vi "Omniax_mDrive_COM8_COM9.vi"() -> ()   [LabVIEW 2009]
uses:
  <vilib>/Instr/_visa.llb/VISA Configure Serial Port (Instr).vi
panel:
  in  "GPIT Backlash":i32
  in  "DETT Backlash":i32
  in  "SY/SZ":dbl max=1.0 step=1.0
  out "GPIT Status":string
  out "read buffer 3":string
  out "SZ":i32
  out "SZ Range?":bool
  out "GPIT rev/sec":dbl caption="Velocity"
  out "GPIT MINPOS":i32=-94296
  out "GPIT MAXPOS":i32=-34296
  out "GPIT COM PORT":refnum<visa-resource-name>="COM5"
  out "SZ Step":i32
  in  "Stop":bool
  out "SY Range?":bool
  out "SY":i32
  out "read buffer 2":string
  out "DETH Status":string
  out "DETH rev//sec":dbl caption="Velocity"
  in  "Go":bool
  in  "SY Step":i32=-1000 min=-1000 max=1000 step=100
  out "DETH MINPOS":i32=-94296
  out "DETH MAXPOS":i32=-34296
  out "DETT COM PORT":refnum<visa-resource-name>="COM5"
  # "SY COM8 & SZ COM9"
  # "20000 steps/rev\n2.5mm/rev\n0.05rev/sec"
  # "20000 steps/rev\n1 mm/rev\n0.01rev/sec"
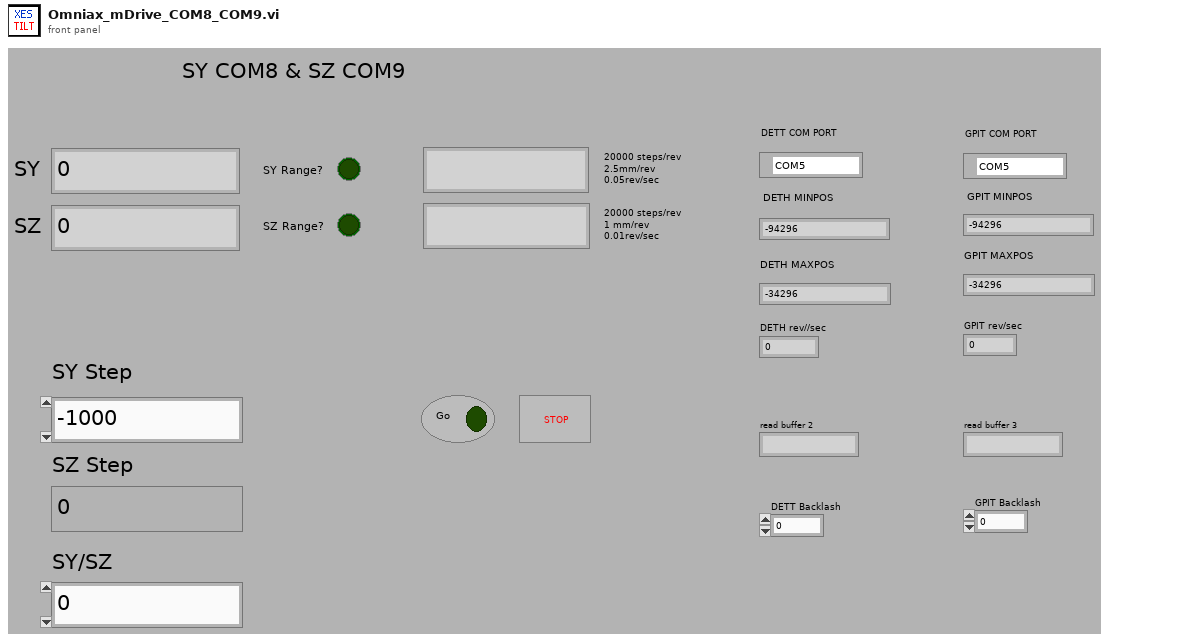
[diagram p1: front panel]
types:
  T1 = enum16{"Stop", "Reset", "Run Current", "Holding Current", "Accel Rate", "Decel Rate", "Move to Relative Position", "Move to Absolute Position", "Prtint Position", "Print Encorder", "Print Velocity", "Microstep Resolution", "Max Velocity"}
  T2 = enum16{"Power-up Signature", "Accel Rate", "Accel Max", "Bit Rate", "Buffer Status", "Change Current", "Commence Jogging", "Change Jog Speed", "Continue", "Define Address", "Distance for FC,FM,FO,FY", "Decel Rate", "Distance or Position", "Define Limits", "Encoder Deadband", "Encoder Function", "Encoder Position", "Encoder Ratio", "Feed to Length with Speed Change", "Feed to Length", "Feed to Sensor with Mask Dist", "Feed to Length & Set Output", "Feed to Position", "Feed to Sensor", "Feed to Sensor w/safety", "Follow Handwheel", "Immediate Distance?", "Immediate Encoder?", "Immediate Low Output", "Immediate High Output", "Immediate Position?", "Input Status?", "Jog Accel/Decel", "Jog Disable", "Jog Enable", "Jog Speed", "Motor Disable", "Motor Enable", "Microstep Resolution", "Power up Current", "Power up Mode", "Pause", "Request Status", "Revision Level?", "Seek Home", "Stop Jogging", "Stop & Kill Buffer", "Set Output", "Set ABS Position", "Send String", "Stop", "Velocity for Speed Change", "Velocity Setting", "Wait for Input", "Wait Time"}
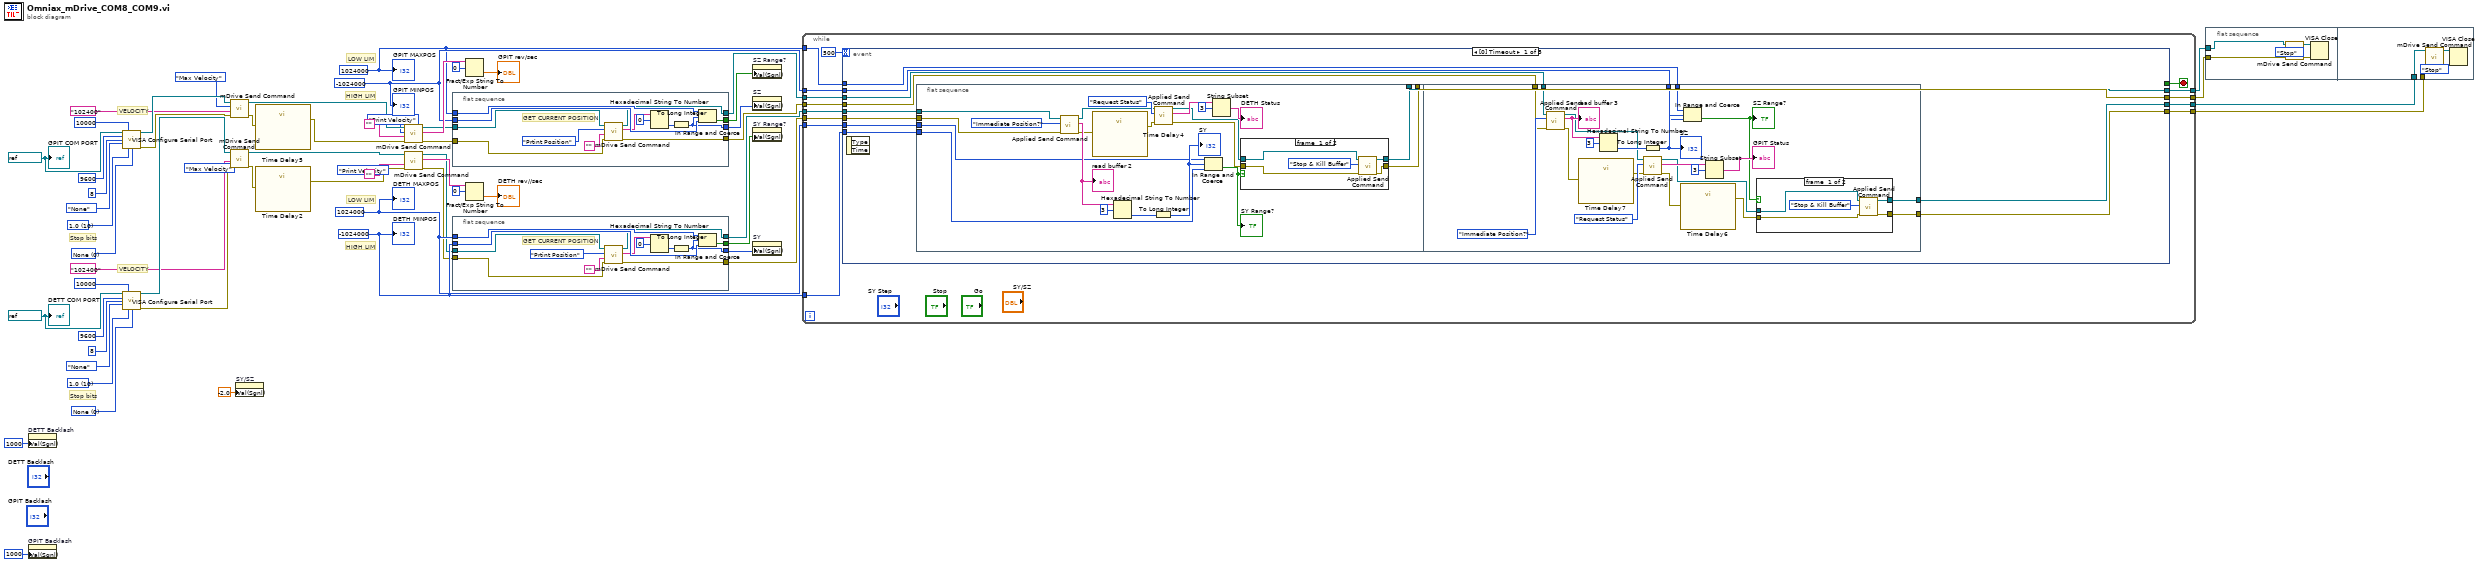
[diagram p0: block diagram]
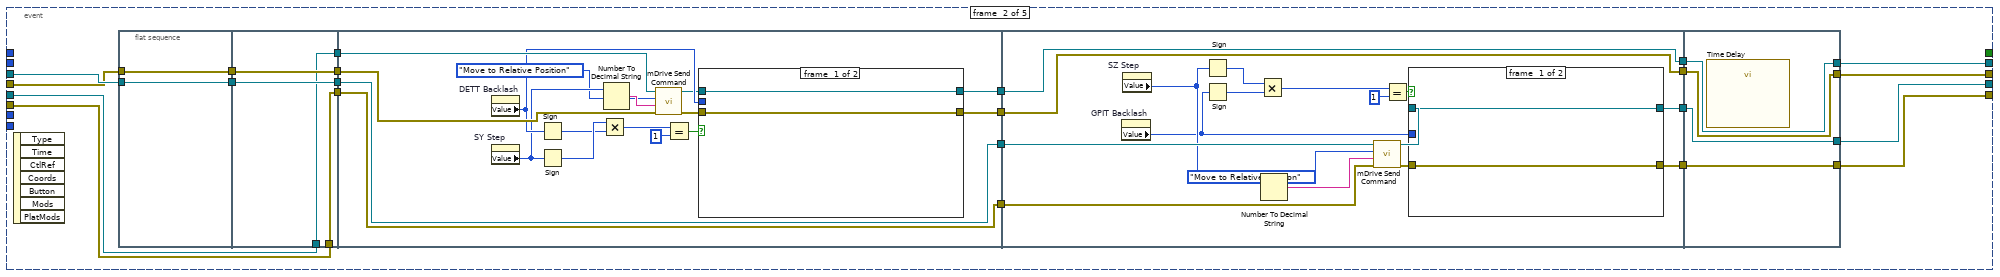
[diagram p4: hidden frame]
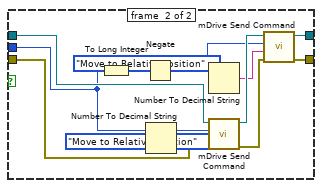
[diagram p5: hidden frame]
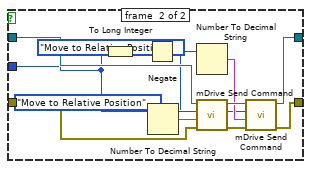
[diagram p6: hidden frame]
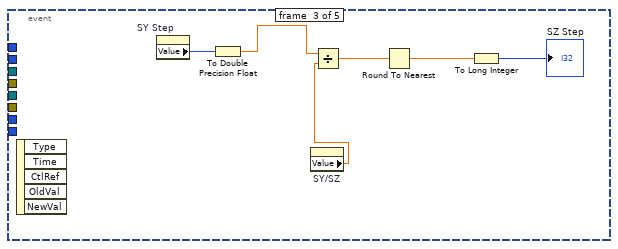
[diagram p7: hidden frame]
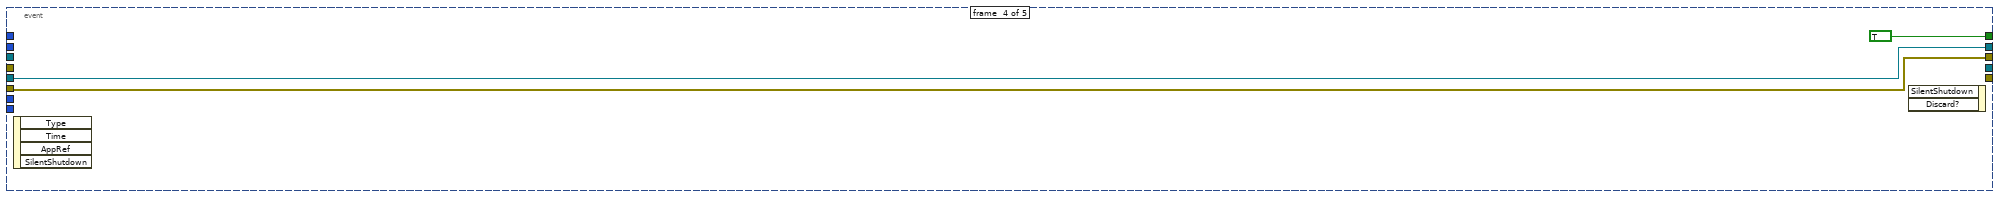
[diagram p8: hidden frame]
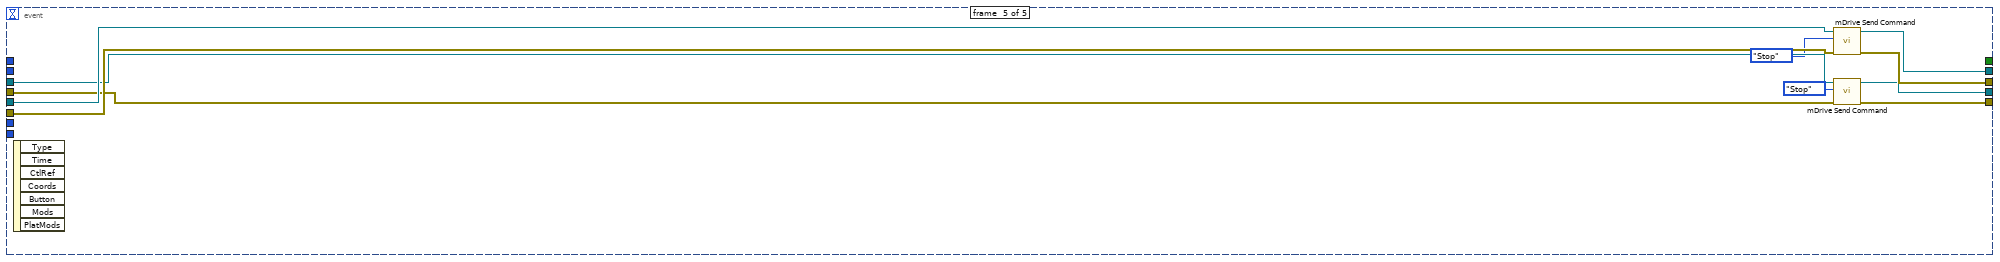
[diagram p9: hidden frame]
diagram:
  w16 = -1024000 ("lower limit")
  w15 = 1024000 ("upper limit")
  w29 = refnum<visa-resource-name> "COM8" ("COM PORT")
  w31 = u16 0 items=["None", "XON/XOFF", "RTS/CTS", "XON/XOFF & RTS/CTS", "DTR/DSR", "XON/XOFF & DTR/DSR"] ("flow control (0:none)")
  w32 = u16 10 items=["1.0"=10, "1.5"=15, "2.0"=20] ("stop bits (10: 1 bit)")
  w51 = -1024000 ("lower limit")
  w52 = 1024000 ("upper limit")
  w55 = refnum<visa-resource-name> "COM9" ("COM PORT")
  w57 = u16 0 items=["None", "XON/XOFF", "RTS/CTS", "XON/XOFF & RTS/CTS", "DTR/DSR", "XON/XOFF & DTR/DSR"] ("flow control (0:none)")
  w58 = u16 10 items=["1.0"=10, "1.5"=15, "2.0"=20] ("stop bits (10: 1 bit)")
  # "VELOCITY"
  # "HIGH LIM"
  # "LOW LIM"
  # "Stop bits"
  # "VELOCITY"
  # "HIGH LIM"
  # "LOW LIM"
  # "Stop bits"
  n1 = property on="DETT Backlash" class="DigNum (strict)"("Val(Sgnl)"=1000 ("Value (Signaling)")) -> ()  [unwired: 2 in, 2 out]
  n2 = property on="GPIT Backlash" class="DigNum (strict)"("Val(Sgnl)"=1000 ("Value (Signaling)")) -> ()  [unwired: 2 in, 2 out]
  n3 = call-poly "VISA Configure Serial Port"("VISA resource name"=w29, "timeout (10sec)"=u32 10000, "baud rate (9600)"=u32 9600, "data bits (8)"=u16 8, "parity (0:none)"=enum16{"None", "Odd", "Even", "Mark", "Space"}."None", "stop bits (10: 1 bit)"=w32, "flow control (0:none)"=w31) -> ("VISA resource name out"=w19:refnum<visa-resource-name>, "error out"=w18:errorcluster)  [unwired: 7 in]
  n4 = call-poly "VISA Configure Serial Port"("VISA resource name"=w55, "timeout (10sec)"=u32 10000, "baud rate (9600)"=u32 9600, "data bits (8)"=u16 8, "parity (0:none)"=enum16{"None", "Odd", "Even", "Mark", "Space"}."None", "stop bits (10: 1 bit)"=w58, "flow control (0:none)"=w57) -> ("VISA resource name out"=w39:refnum<visa-resource-name>, "error out"=w38:errorcluster)  [unwired: 7 in]
  n5 = call "mDrive Send Command.vi"("error in (no error)"=w18, "Extra"="102400", "Command"=T1."Max Velocity", "VISA resource name"=w19) -> ("error out"=w28:errorcluster, "VISA resource name out"=w24:refnum<visa-resource-name>)  [unwired: 3 in, 1 out]
  n6 = call "mDrive Send Command.vi"("error in (no error)"=w38, "Extra"="102400", "Command"=T1."Max Velocity", "VISA resource name"=w39) -> ("error out"=w50:errorcluster, "VISA resource name out"=w46:refnum<visa-resource-name>)  [unwired: 3 in, 1 out]
  n7 = property on="SY/SZ" class="DigNum (strict)"("Val(Sgnl)"=-2.0 ("Value (Signaling)")) -> ()  [unwired: 2 in, 2 out]
  n8 = call "Time Delay5"("error in (no error)"=w28) -> ("error out"=w25:errorcluster)  [unwired: 10 in]
  n9 = call "Time Delay2"("error in (no error)"=w50) -> ("error out"=w47:errorcluster)  [unwired: 10 in]
  n10 = call "mDrive Send Command.vi"("error in (no error)"=w25, "Extra"="", "Command"=T1."Print Velocity", "VISA resource name"=w24) -> ("error out"=w22:errorcluster, "read buffer"=w27:string, "VISA resource name out"=w23:refnum<visa-resource-name>)  [unwired: 3 in]
  n11 = call "mDrive Send Command.vi"("error in (no error)"=w47, "Extra"="", "Command"=T1."Print Velocity", "VISA resource name"=w46) -> ("error out"=w44:errorcluster, "read buffer"=w49:string, "VISA resource name out"=w45:refnum<visa-resource-name>)  [unwired: 3 in]
  n12 = flat-sequence {
    tunnel: w22 -> [w74]
    tunnel: w23 -> [w73]
    tunnel: w15 -> [w71]
    tunnel: w16 -> [w70]
    tunnel: [w72] -> w13
    tunnel: [w63] -> w8
    tunnel: [w69] -> w10
    tunnel: [w68] -> w14
    frame #0 {
      # "GET CURRENT POSITION"
      n13 = call "mDrive Send Command.vi"("error in (no error)"=w74, "Extra"="", "Command"=T1."Prtint Position", "VISA resource name"=w73) -> ("error out"=w72:errorcluster, "read buffer"=w66:string, "VISA resource name out"=w68:refnum<visa-resource-name>)  [unwired: 3 in]
      n14 = Hexadecimal String To Number(string=w66, offset=0) -> (number=w64:u32)  [unwired: 1 in, 1 out]
      n15 = To Long Integer(number=w64) -> (32bit integer=w63:i32)
      n16 = In Range and Coerce(upper limit=w71, x=w63, lower limit=w70) -> (In Range?=w69:bool)  [unwired: 1 out]
    }
  }
  n17 = flat-sequence {
    tunnel: w44 -> [w87]
    tunnel: w45 -> [w86]
    tunnel: w52 -> [w85]
    tunnel: w51 -> [w84]
    tunnel: [w76] -> w53
    tunnel: [w77] -> w9
    tunnel: [w83] -> w36
    tunnel: [w82] -> w54
    frame #0 {
      # "GET CURRENT POSITION"
      n18 = call "mDrive Send Command.vi"("error in (no error)"=w87, "Extra"="", "Command"=T1."Prtint Position", "VISA resource name"=w86) -> ("error out"=w76:errorcluster, "read buffer"=w80:string, "VISA resource name out"=w82:refnum<visa-resource-name>)  [unwired: 3 in]
      n19 = Hexadecimal String To Number(string=w80, offset=0) -> (number=w78:u32)  [unwired: 1 in, 1 out]
      n20 = To Long Integer(number=w78) -> (32bit integer=w77:i32)
      n21 = In Range and Coerce(upper limit=w85, x=w77, lower limit=w84) -> (In Range?=w83:bool)  [unwired: 1 out]
    }
  }
  n22 = Fract/Exp String To Number(string=w27, offset=0) -> (number=→"GPIT rev/sec":dbl)  [unwired: 2 in, 1 out]
  n23 = Fract/Exp String To Number(string=w49, offset=0) -> (number=→"DETH rev//sec":dbl)  [unwired: 2 in, 1 out]
  n24 = property on="SZ Range?" class="Bool (strict)"("Val(Sgnl)"=w10) -> ()  [unwired: 2 in, 2 out]
  n25 = property on="SZ" class="DigNum (strict)"("Val(Sgnl)"=w8) -> ()  [unwired: 2 in, 2 out]
  n26 = property on="SY Range?" class="Bool (strict)"("Val(Sgnl)"=w36) -> ()  [unwired: 2 in, 2 out]
  n27 = property on="SY" class="DigNum (strict)"("Val(Sgnl)"=w9) -> ()  [unwired: 2 in, 2 out]
  n28 = while {
    tunnel: w54 -> [w95]
    tunnel: w53 -> [w100]
    tunnel: [w101] -> w40
    tunnel: [w99] -> w41
    tunnel: w52 -> [w98]
    tunnel: w51 -> [w97]
    tunnel: w16 -> [w93]
    tunnel: w15 -> [w88]
    tunnel: w14 -> [w92]
    tunnel: w13 -> [w91]
    tunnel: [w90] -> w12
    tunnel: [w89] -> w11
    stop <- w94 stop-if-true
    n29 = event shown="[0] Timeout" {
      selector: _ -> [_ _ _ _ _]
      dyn-events: _ -> [_ _ _ _ _]
      timeout: 500 -> [_ _ _ _ _]
      tunnel: w100 -> [w111 w172 _ w274 w284]
      tunnel: [w105 w179 _ w274 w282] -> w101
      tunnel: w95 -> [w110 w171 _ w275 w285]
      tunnel: [w104 w192 _ w275 w283] -> w99
      tunnel: w98 -> [w113 _ _ _ _]
      tunnel: w97 -> [w112 _ _ _ _]
      tunnel: [_ _ _ TRUE _] -> w94
      tunnel: w93 -> [w102 _ _ _ _]
      tunnel: w88 -> [w103 _ _ _ _]
      tunnel: w92 -> [w109 w187 _ _ w279]
      tunnel: w91 -> [w108 w183 _ _ w278]
      tunnel: [w107 w177 _ _ w281] -> w90
      tunnel: [w106 w175 _ _ w280] -> w89
      event #0 {
        n30 = event-data() -> ()  [unwired: 1 in, 2 out]
        n31 = flat-sequence {
          tunnel: w112 -> [w134]
          tunnel: w113 -> [w126]
          tunnel: w111 -> [w125]
          tunnel: w110 -> [w124]
          tunnel: [w116] -> w104
          tunnel: [w114] -> w105
          tunnel: w109 -> [w150]
          tunnel: w108 -> [w149]
          tunnel: w103 -> [w148]
          tunnel: w102 -> [w147]
          tunnel: [w144] -> w107
          tunnel: [w145] -> w106
          frame #0 {
            n32 = call "Applied Send Command.vi"("error in (no error)"=w125, "Command"=T2."Immediate Position?", "VISA resource name"=w124) -> ("error out"=w120:errorcluster, "read buffer"=w132:string, "VISA resource name out"=w127:refnum<visa-resource-name>)  [unwired: 4 in]
            "read buffer 2" <- w132
            n33 = call "Time Delay4"("error in (no error)"=w120) -> ("error out"=w119:errorcluster)  [unwired: 10 in]
            n34 = Hexadecimal String To Number(string=w132, offset=3) -> (number=w131:u32)  [unwired: 1 in, 1 out]
            n35 = call "Applied Send Command.vi"("error in (no error)"=w119, "Command"=T2."Request Status", "VISA resource name"=w127) -> ("error out"=w115:errorcluster, "read buffer"=w123:string, "VISA resource name out"=w117:refnum<visa-resource-name>)  [unwired: 4 in]
            n36 = To Long Integer(number=w131) -> (32bit integer=w129:i32)
            "SY" <- w129
            n37 = In Range and Coerce(upper limit=w126, x=w129, lower limit=w134) -> (In Range?=w118:bool)  [unwired: 1 out]
            "SY Range?" <- w118
            n38 = String Subset(string=w123, offset (0)=3) -> (substring=→"DETH Status":string)  [unwired: 1 in]
            n39 = case shown="False" w118 {
              tunnel: w117 -> [w136 w141]
              tunnel: [w138 w141] -> w116
              tunnel: [w139 w140] -> w114
              tunnel: w115 -> [w135 w140]
              frame #0 {
                n40 = call "Applied Send Command.vi"("error in (no error)"=w135, "Command"=T2."Stop & Kill Buffer", "VISA resource name"=w136) -> ("error out"=w139:errorcluster, "VISA resource name out"=w138:refnum<visa-resource-name>)  [unwired: 4 in, 1 out]
              }
              frame #1 {
              }
            }
          }
          frame #1 {
            n41 = call "Applied Send Command.vi"("error in (no error)"=w149, "Command"=T2."Immediate Position?", "VISA resource name"=w150) -> ("error out"=w152:errorcluster, "read buffer"=w162:string, "VISA resource name out"=w157:refnum<visa-resource-name>)  [unwired: 4 in]
            "read buffer 3" <- w162
            n42 = call "Time Delay7"("error in (no error)"=w152) -> ("error out"=w151:errorcluster)  [unwired: 10 in]
            n43 = Hexadecimal String To Number(string=w162, offset=3) -> (number=w161:u32)  [unwired: 1 in, 1 out]
            n44 = To Long Integer(number=w161) -> (32bit integer=w159:i32)
            "SZ" <- w159
            n45 = call "Applied Send Command.vi"("error in (no error)"=w151, "Command"=T2."Request Status", "VISA resource name"=w157) -> ("error out"=w156:errorcluster, "read buffer"=w155:string, "VISA resource name out"=w143:refnum<visa-resource-name>)  [unwired: 4 in]
            n46 = call "Time Delay6"("error in (no error)"=w156) -> ("error out"=w146:errorcluster)  [unwired: 10 in]
            n47 = In Range and Coerce(upper limit=w148, x=w159, lower limit=w147) -> (In Range?=w142:bool)  [unwired: 1 out]
            "SZ Range?" <- w142
            n48 = String Subset(string=w155, offset (0)=3) -> (substring=→"GPIT Status":string)  [unwired: 1 in]
            n49 = case shown="False" w142 {
              tunnel: w143 -> [w165 w170]
              tunnel: [w167 w170] -> w144
              tunnel: [w168 w169] -> w145
              tunnel: w146 -> [w164 w169]
              frame #0 {
                n50 = call "Applied Send Command.vi"("error in (no error)"=w164, "Command"=T2."Stop & Kill Buffer", "VISA resource name"=w165) -> ("error out"=w168:errorcluster, "VISA resource name out"=w167:refnum<visa-resource-name>)  [unwired: 4 in, 1 out]
              }
              frame #1 {
              }
            }
          }
        }
      }
      event #1 {
        n51 = event-data() -> ()  [unwired: 1 in, 7 out]
        n52 = flat-sequence {
          tunnel: w187 -> [w194]
          tunnel: [w194] -> w186
          tunnel: [w193] -> w184
          tunnel: w183 -> [w193]
          tunnel: [w198] -> w189
          tunnel: w186 -> [w198]
          tunnel: [w197] -> w185
          tunnel: w184 -> [w197]
          tunnel: [w196] -> w174
          tunnel: [w195] -> w173
          tunnel: w172 -> [w195]
          tunnel: w171 -> [w196]
          tunnel: [w201] -> w191
          tunnel: w189 -> [w215]
          tunnel: [w215] -> w188
          tunnel: w185 -> [w213]
          tunnel: [w212] -> w182
          tunnel: [w200] -> w181
          tunnel: w174 -> [w214]
          tunnel: w173 -> [w212]
          tunnel: w191 -> [w247]
          tunnel: [w247] -> w190
          tunnel: w188 -> [w246]
          tunnel: w182 -> [w245]
          tunnel: w181 -> [w244]
          tunnel: [w244] -> w180
          tunnel: [w232] -> w178
          tunnel: [w234] -> w176
          tunnel: [w266] -> w192
          tunnel: w190 -> [w266]
          tunnel: w180 -> [w265]
          tunnel: [w265] -> w179
          tunnel: w178 -> [w264]
          tunnel: [w264] -> w177
          tunnel: [w263] -> w175
          tunnel: w176 -> [w263]
          frame #0 {
          }
          frame #1 {
          }
          frame #2 {
            n53 = property on="DETT Backlash" class="DigNum (strict)"() -> ("Value"=w205:i32)  [unwired: 2 in, 2 out]
            n54 = property on="SY Step" class="DigNum (strict)"() -> ("Value"=w204:i32)  [unwired: 2 in, 2 out]
            n55 = Sign(1:w205) -> (0:w209:i32)
            n56 = Sign(1:w204) -> (0:w210:i32)
            n57 = Multiply(x=w210, y=w209) -> (x*y=w208:i32)
            n58 = Number To Decimal String(number=w204) -> (decimal integer string=w211:string)  [unwired: 1 in]
            n59 = call "mDrive Send Command.vi"("error in (no error)"=w213, "Extra"=w211, "Command"=T1."Move to Relative Position", "VISA resource name"=w214) -> ("error out"=w202:errorcluster, "VISA resource name out"=w203:refnum<visa-resource-name>)  [unwired: 3 in, 1 out]
            n60 = Equal?(x=w208, y=1) -> (x = y?=w206:bool)
            n61 = case shown="True" w206 {
              tunnel: w203 -> [w217 w230]
              tunnel: [w217 w224] -> w201
              tunnel: [w216 w225] -> w200
              tunnel: w202 -> [w216 w229]
              tunnel: w205 -> [_ w220]
              frame #0 {
              }
              frame #1 {
                n62 = To Long Integer(number=w220) -> (32bit integer=w222:i32)
                n63 = Negate(x=w222) -> (-x=w223:i32)
                n64 = Number To Decimal String(number=w220) -> (decimal integer string=w228:string)  [unwired: 1 in]
                n65 = Number To Decimal String(number=w223) -> (decimal integer string=w221:string)  [unwired: 1 in]
                n66 = call "mDrive Send Command.vi"("error in (no error)"=w229, "Extra"=w228, "Command"=T1."Move to Relative Position", "VISA resource name"=w230) -> ("error out"=w226:errorcluster, "VISA resource name out"=w227:refnum<visa-resource-name>)  [unwired: 3 in, 1 out]
                n67 = call "mDrive Send Command.vi"("error in (no error)"=w226, "Extra"=w221, "Command"=T1."Move to Relative Position", "VISA resource name"=w227) -> ("error out"=w225:errorcluster, "VISA resource name out"=w224:refnum<visa-resource-name>)  [unwired: 3 in, 1 out]
              }
            }
          }
          frame #3 {
            n68 = property on="GPIT Backlash" class="DigNum (strict)"() -> ("Value"=w236:i32)  [unwired: 2 in, 2 out]
            n69 = property on="SZ Step" class="DigNum (strict)"() -> ("Value"=w238:i32)  [unwired: 2 in, 2 out]
            n70 = Sign(1:w238) -> (0:w242:i32)
            n71 = Sign(1:w236) -> (0:w241:i32)
            n72 = Multiply(x=w242, y=w241) -> (x*y=w240:i32)
            n73 = Number To Decimal String(number=w238) -> (decimal integer string=w243:string)  [unwired: 1 in]
            n74 = call "mDrive Send Command.vi"("error in (no error)"=w245, "Extra"=w243, "Command"=T1."Move to Relative Position", "VISA resource name"=w246) -> ("error out"=w235:errorcluster, "VISA resource name out"=w233:refnum<visa-resource-name>)  [unwired: 3 in, 1 out]
            n75 = Equal?(x=w240, y=1) -> (x = y?=w237:bool)
            n76 = case shown="True" w237 {
              tunnel: w233 -> [w249 w262]
              tunnel: [w249 w256] -> w232
              tunnel: [w248 w257] -> w234
              tunnel: w235 -> [w248 w261]
              tunnel: w236 -> [_ w252]
              frame #0 {
              }
              frame #1 {
                n77 = To Long Integer(number=w252) -> (32bit integer=w254:i32)
                n78 = Negate(x=w254) -> (-x=w255:i32)
                n79 = Number To Decimal String(number=w252) -> (decimal integer string=w260:string)  [unwired: 1 in]
                n80 = Number To Decimal String(number=w255) -> (decimal integer string=w253:string)  [unwired: 1 in]
                n81 = call "mDrive Send Command.vi"("error in (no error)"=w261, "Extra"=w260, "Command"=T1."Move to Relative Position", "VISA resource name"=w262) -> ("error out"=w258:errorcluster, "VISA resource name out"=w259:refnum<visa-resource-name>)  [unwired: 3 in, 1 out]
                n82 = call "mDrive Send Command.vi"("error in (no error)"=w258, "Extra"=w253, "Command"=T1."Move to Relative Position", "VISA resource name"=w259) -> ("error out"=w257:errorcluster, "VISA resource name out"=w256:refnum<visa-resource-name>)  [unwired: 3 in, 1 out]
              }
            }
          }
          frame #4 {
            n83 = call "Time Delay"() -> ()  [unwired: 11 in, 1 out]
          }
        }
      }
      event #2 {
        n84 = event-data() -> ()  [unwired: 1 in, 5 out]
        n85 = property on="SY Step" class="DigNum (strict)"() -> ("Value"=w268:i32)  [unwired: 2 in, 2 out]
        n86 = To Double Precision Float(number=w268) -> (double precision float=w269:dbl)
        n87 = property on="SY/SZ" class="DigNum (strict)"() -> ("Value"=w267:dbl)  [unwired: 2 in, 2 out]
        n88 = Divide(x=w269, y=w267) -> (x/y=w272:dbl)
        n89 = Round To Nearest(number=w272) -> (nearest integer value=w271:dbl)
        n90 = To Long Integer(number=w271) -> (32bit integer=→"SZ Step":i32)
      }
      event #3 {
        n91 = event-data() -> ()  [unwired: 1 in, 4 out]
        n92 = event-data() -> ()  [unwired: 3 in, 1 out]
      }
      event #4 {
        n93 = event-data() -> ()  [unwired: 1 in, 7 out]
        n94 = call "mDrive Send Command.vi"("error in (no error)"=w284, "Command"=T1."Stop", "VISA resource name"=w285) -> ("error out"=w282:errorcluster, "VISA resource name out"=w283:refnum<visa-resource-name>)  [unwired: 4 in, 1 out]
        n95 = call "mDrive Send Command.vi"("error in (no error)"=w278, "Command"=T1."Stop", "VISA resource name"=w279) -> ("error out"=w280:errorcluster, "VISA resource name out"=w281:refnum<visa-resource-name>)  [unwired: 4 in, 1 out]
      }
    }
  }
  n96 = flat-sequence {
    tunnel: w41 -> [w290]
    tunnel: w40 -> [w287]
    tunnel: w12 -> [w292]
    tunnel: w11 -> [w293]
    frame #0 {
      n97 = call "mDrive Send Command.vi"("error in (no error)"=w287, "Command"=T1."Stop", "VISA resource name"=w290) -> ("error out"=w288:errorcluster, "VISA resource name out"=w289:refnum<visa-resource-name>)  [unwired: 4 in, 1 out]
      n98 = VISA Close(VISA resource name=w289, error in (no error)=w288) -> ()  [unwired: 1 out]
    }
    frame #1 {
      n99 = call "mDrive Send Command.vi"("error in (no error)"=w293, "Command"=T1."Stop", "VISA resource name"=w292) -> ("error out"=w294:errorcluster, "VISA resource name out"=w295:refnum<visa-resource-name>)  [unwired: 4 in, 1 out]
      n100 = VISA Close(VISA resource name=w295, error in (no error)=w294) -> ()  [unwired: 1 out]
    }
  }
  "DETT COM PORT" <- w55
  "DETH MAXPOS" <- w52
  "DETH MINPOS" <- w51
  "GPIT COM PORT" <- w29
  "GPIT MAXPOS" <- w15
  "GPIT MINPOS" <- w16
